vi "TestStand.ReportErrorCallback.vi"(4 "state variables in":T1={"DUTs.Name"=["All", "Station 1", "Station 2", "Station 3"], "Pages.Name"=[], "Pages.Ref"=[], "TS.UI"={"References"={"Event Callback"=refnum, "Quit Application Event"=refnum, "Events"=refnum, "Top level VI"=refnum, "TestStand Engine"=refnum, "Start Application Event"=refnum, "Stop Application Event"=refnum}, "Managers"={"Application Manager"=refnum, "SequenceFileView Manager"=refnum, "ExecutionView Manager"=refnum}, "Controls"={"Execution View"=refnum, "Run Button"=refnum, "Open Button"=refnum}}, "TS.Running"=FALSE, "TS.Abort"=FALSE, "NIVS.GatewayIPAddress"="", "NIVS.WorkspaceManager"=refnum, "NIVS.Open"=FALSE, "NIVS.Deployed"=FALSE, "NIVS.SystemStateRefs"={"CustDatRef"=refnum, "EvtRef"=refnum, "Target State User Event"=refnum}, "NIVS.Events"={"SystemChangeEvent"=refnum, "WorkspaceEvent"=refnum}, "UI.Tree"=refnum, "UI.Path"=refnum, "UI.Stop"=refnum, "UI.Tab"=refnum}, 5 "Event data":cluster{"errorCode":i32, "errorMessage":string}, 6 "CtlRef":refnum<k7>, 7 "Event common data":cluster{"Source":i32, "Type":u32, "Time":u32}) -> ()   [LabVIEW 2015, in "Main.GUI.lvlib"]
doc: "The Application Manager generates the ReportError event when TestStand generates an error."
uses:
  Main.GUI.lvlib
  Types/Multihead.StateVariables.ctl
  Types/TestStandGUI.Refs.ctl
  <vilib>/NI Veristand/Execution/Workspace/WorkspaceAPI.ctl
  NationalInstruments.VeriStand.ClientAPI
  <vilib>/NI Veristand/Execution/Workspace/SystemStateEventRef.ctl
  <vilib>/NI Veristand/Execution/Workspace/Target State Info.ctl
  <vilib>/NI Veristand/Execution/Workspace/Target State.ctl
  Execution GUI/Types/Execute.UserEventRefs.ctl
  <vilib>/NI Veristand/Execution/Workspace/SystemStateRegEventRef.ctl
  <vilib>/NI Veristand/Execution/Workspace/NI_VS Workspace ExecutionAPI.lvlib
  Execution GUI/Station.Execution.lvlib
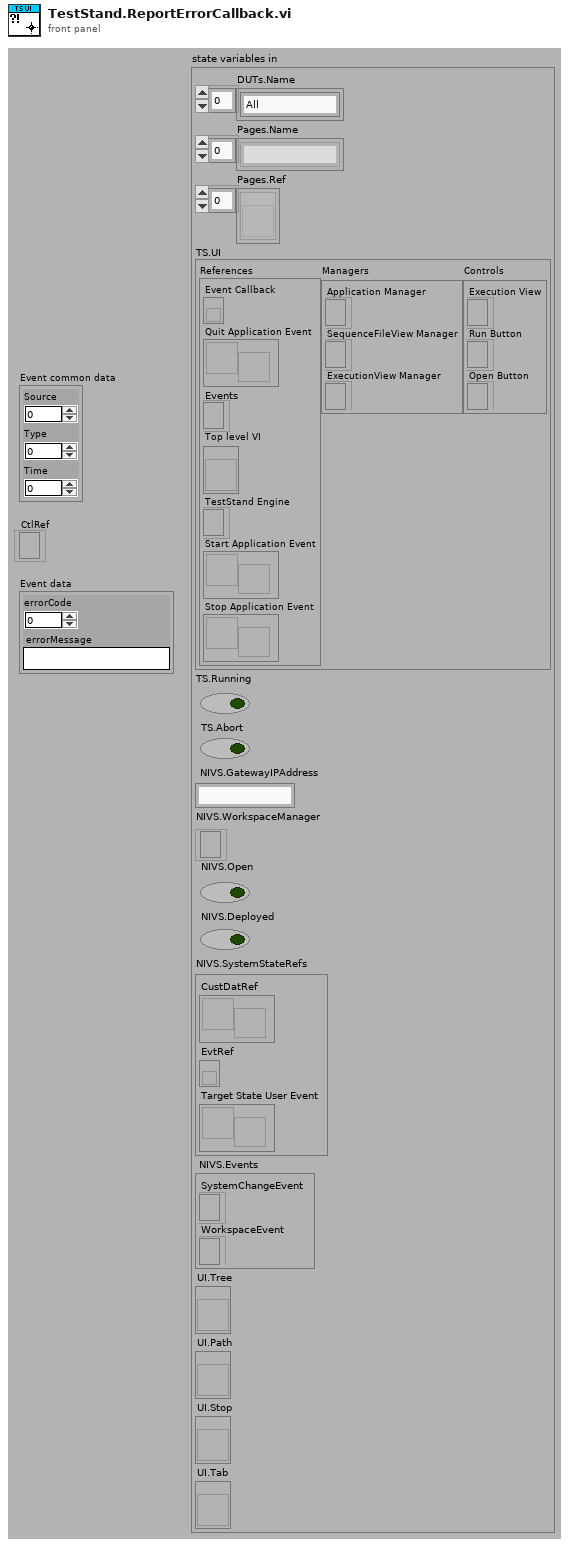
[diagram p1: front panel]
types:
  T1 = typedef "Main.GUI.lvlib/Multihead.StateVariables.ctl" = cluster{"DUTs.Name":string[], "Pages.Name":string[], "Pages.Ref":refnum<vi>[], "TS.UI":T2, "TS.Running":bool, "TS.Abort":bool, "NIVS.GatewayIPAddress":string, "NIVS.WorkspaceManager":T3, "NIVS.Open":bool, "NIVS.Deployed":bool, "NIVS.SystemStateRefs":T4, "NIVS.Events":T5, "UI.Tree":refnum<vi>, "UI.Path":refnum<vi>, "UI.Stop":refnum<vi>, "UI.Tab":refnum<vi>}
  T2 = typedef "Main.GUI.lvlib/TestStandGUI.Refs.ctl" = cluster{"References":cluster{"Event Callback":refnum<k27>, "Quit Application Event":refnum<user-event>, "Events":refnum<event-registration>, "Top level VI":refnum<vi>, "TestStand Engine":refnum<k7>, "Start Application Event":refnum<user-event>, "Stop Application Event":refnum<user-event>}, "Managers":cluster{"Application Manager":refnum<k7>, "SequenceFileView Manager":refnum<k7>, "ExecutionView Manager":refnum<k7>}, "Controls":cluster{"Execution View":refnum<k7>, "Run Button":refnum<k7>, "Open Button":refnum<k7>}}
  T3 = typedef "NI_VS Workspace ExecutionAPI.lvlib/WorkspaceAPI.ctl" = refnum<k24>
  T4 = typedef "NI_VS Workspace ExecutionAPI.lvlib/SystemStateEventRef.ctl" = cluster{"CustDatRef":refnum<user-event>, "EvtRef":refnum<k27>, "Target State User Event":refnum<user-event>}
  T5 = typedef "Station.Execution.lvlib/Execute.UserEventRefs.ctl" = cluster{"SystemChangeEvent":T6, "WorkspaceEvent":refnum<event-registration>}
  T6 = typedef "NI_VS Workspace ExecutionAPI.lvlib/SystemStateRegEventRef.ctl" = refnum<event-registration>
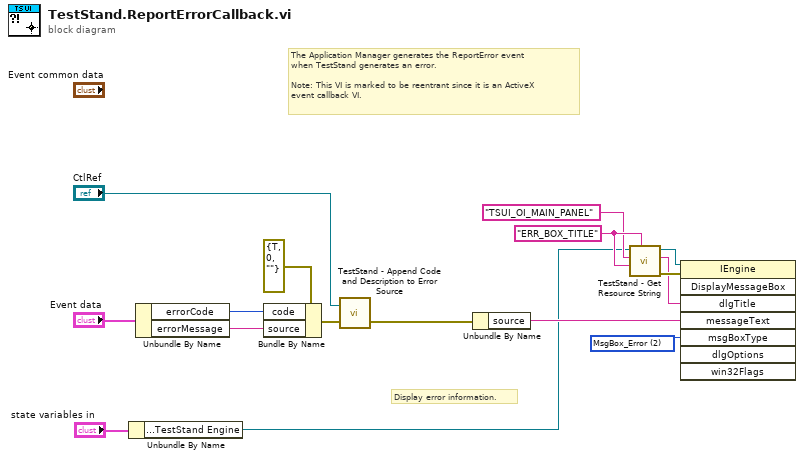
[diagram p0: block diagram]
diagram:
  w5 = 2 items=["MsgBox_Warning", "MsgBox_Information", "MsgBox_Error", "MsgBox_Custom"] ("msgBoxType")
  w8 = "ERR_BOX_TITLE" ("Symbol")
  # "Display error information."
  # "The Application Manager generates the ReportError event\nwhen TestStand generates an error.\n\nNote: This VI is marked to be reentrant since it is an ActiveX\nevent callback VI."
  n1 = Unbundle By Name("state variables in") -> ("TS.UI.References.TestStand Engine"=w1:refnum<k7>)
  n2 = Unbundle By Name("Event data") -> ("errorCode"=w14:i32, "errorMessage"=w15:string)
  n3 = Bundle By Name(cluster=errorcluster {"status"=TRUE, "code"=0, "source"=""} ("error in (no error)"), "code"=w14, "source"=w15) -> (w12:errorcluster)
  n4 = call <vilib>:"TestStand - Append Code and Description to Error Source.vi"("error in (no error)"=w12, "Application Manager Ref In"="CtlRef") -> ("error out"=w4:errorcluster)  [unwired: 1 out]
  n5 = Unbundle By Name(w4) -> ("source"=w6:string)
  n6 = call <vilib>:"TestStand - Get Resource String.vi"("Default String"=w8, "Symbol"=w8, "Category"="TSUI_OI_MAIN_PANEL", "Engine Reference In"=w1) -> ("error out"=w11:errorcluster, "Resource String"=w9:string, "Engine Reference Out"=w10:refnum<k7>)  [unwired: 1 in, 4 out]
  n7 = invoke class="IEngine" method="DisplayMessageBox"(reference=w10, error in=w11, "dlgTitle"=w9, "messageText"=w6, "msgBoxType"=w5) -> ()  [unwired: 3 in, 8 out]
